vi "Write Time domain analyzer class.vi"(10 "Instrument.lvclass":refnum<class "Instrument.lvclass">, 11 "Switching Time in":refnum<class "Switching Time.lvclass">) -> (3 "Switching Time out":refnum<class "Switching Time.lvclass">)   [LabVIEW 2020, in "Switching Time.lvclass"]
uses:
  Switching Time.lvclass
  Instruments/Instrument.lvclass
  Switching Time.lvclass/Switching Time.ctl
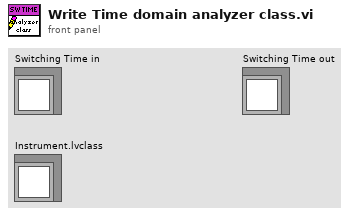
[diagram p1: front panel]
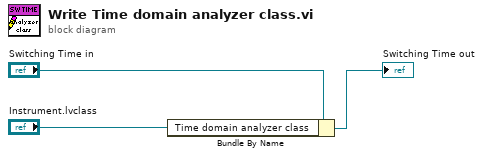
[diagram p0: block diagram]
diagram:
  n1 = Bundle By Name(cluster="Switching Time in", "Time domain analyzer class"="Instrument.lvclass") -> (→"Switching Time out":refnum<class "Switching Time.lvclass">)
